vi "FSK.vi"() -> ()   [LabVIEW 2012]
uses:
  <vilib>/express/express analysis/Spectral/Block/exnSpectralBlock spectral measurements peak poly.vi
  <vilib>/express/express analysis/Spectral/Block/exnSpectralBlock spectral measurements peak DDT.vi
  <vilib>/express/express analysis/Spectral/XNode/ExpressSpectralMeasurementsBlockNode.xnode
panel:
  in  "stop":bool
  in  "Slow":dbl
  in  "Fast":dbl
  out "Waveform Graph 2":dynamicdata(graph)
  out "Waveform Graph":dynamicdata(graph)
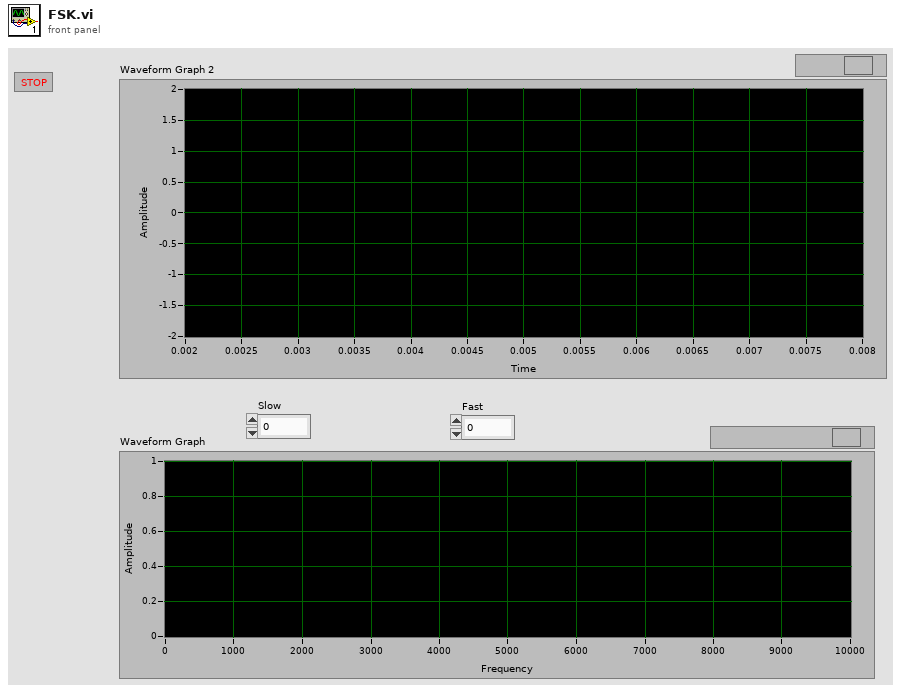
[diagram p1: front panel]
types:
  T1 = cluster{"averaging mode":u16, "weighting mode":u16, "number of averages":u32}
  T2 = cluster{"dB On (F)":bool, "unwrap phase (F)":bool, "convert to degree (F)":bool}
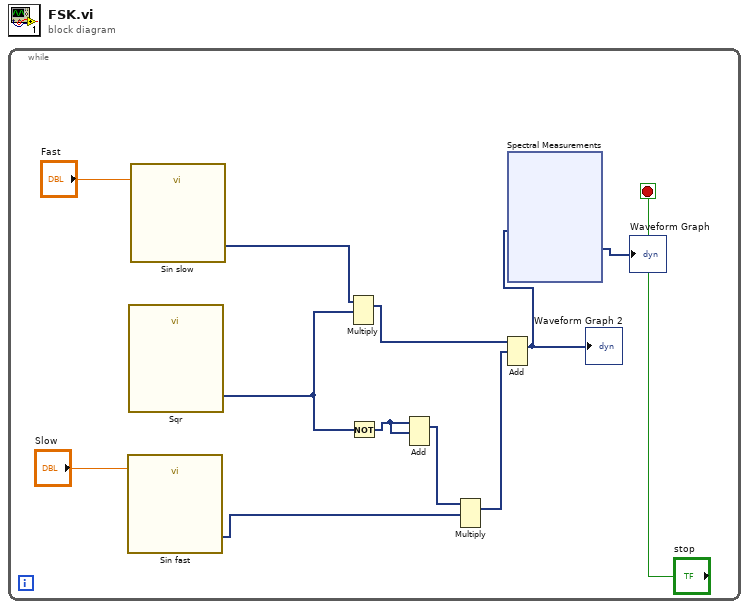
[diagram p0: block diagram]
diagram:
  n1 = while {
    stop <- "stop" stop-if-true
    n2 = call "Sin fast"("Frequency"="Slow") -> ("Sine"=w10:dynamicdata)  [unwired: 13 in, 1 out]
    n3 = call "Sqr"() -> ("Square"=w11:dynamicdata)  [unwired: 14 in, 1 out]
    n4 = call "Sin slow"("Frequency"="Fast") -> ("Sine"=w12:dynamicdata)  [unwired: 13 in, 1 out]
    n5 = Multiply(1:w11, 2:w12) -> (0:w9:dynamicdata)  [unwired: 1 in, 1 out]
    n6 = Not(x=w11) -> (.not. x?=w3:dynamicdata)
    n7 = Add(1:w3, 2:w3) -> (0:w2:dynamicdata)  [unwired: 1 in, 1 out]
    n8 = Multiply(1:w10, 2:w2) -> (0:w4:dynamicdata)  [unwired: 1 in, 1 out]
    n9 = Add(1:w4, 2:w9) -> (0:w7:dynamicdata)  [unwired: 1 in, 1 out]
    "Waveform Graph 2" <- w7
    n10 = xnode "Spectral Measurements"("Signals"=w7) -> ("FFT - (Peak)"=→"Waveform Graph":dynamicdata)  [unwired: 1 in, 2 out]
  }
